vi "test_mzi_fft.vi"() -> ()   [LabVIEW 2009]
doc: "Copyright (c) 2010 Stepan A. Baranov (stepan@baranov.su)\nAll rights reserved.\nweb-site: www.OCTLab.org"
uses:
  <vilib>/Analysis/4window.llb/Hanning Window (DBL).vi
  <vilib>/Analysis/NI_AALPro.lvlib
  OCTLib_64.dll
panel:
  out "error out":errorcluster
  out "Im part":dbl[](array[numeric])
  out "Re part":dbl[](array[numeric])
  out "Phase A-scan":dbl[](array[numeric])
  out "Intensity A-scan":dbl[](array[numeric])
  out "Im":dbl[](array[numeric])
  out "Re":dbl[](array[numeric])
  out "phase":dbl[](array[numeric])
  out "intensity":dbl[](array[numeric])
  out "time for FFT":u32
  in  "RSM_STAT?":bool=TRUE
  in  "stop":bool
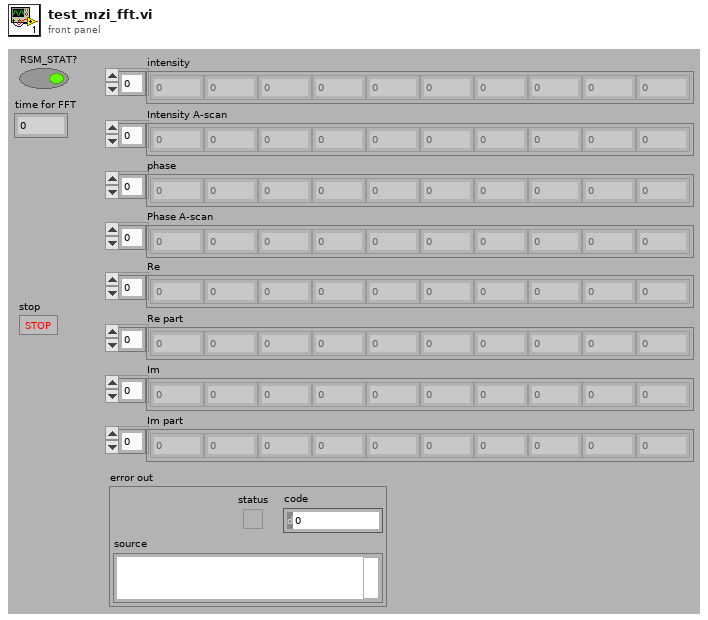
[diagram p1: front panel]
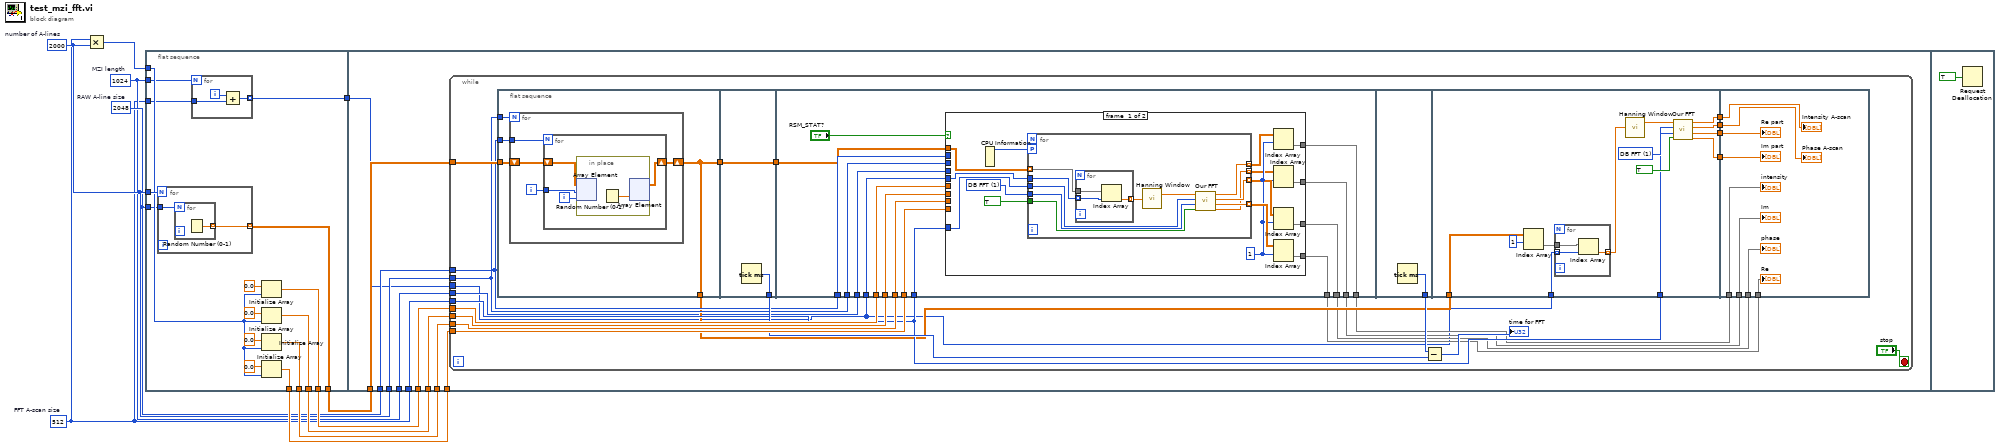
[diagram p0: block diagram]
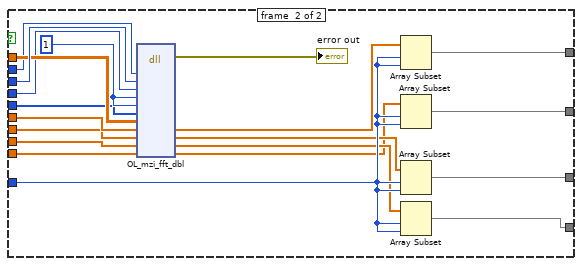
[diagram p2: hidden frame]
diagram:
  w2 = 1024  # MZI length
  w1 = 512  # FFT A-scan size
  w5 = 2000  # number of A-lines
  w4 = 2048  # RAW A-line size
  n1 = Multiply(x=w1, y=w5) -> (x*y=w11:i32)
  n2 = flat-sequence {
    tunnel: w4 -> [w15]
    tunnel: w5 -> [w26]
    tunnel: w11 -> [w21]
    tunnel: [w20] -> w10
    tunnel: [w19] -> w9
    tunnel: [w18] -> w8
    tunnel: [w17] -> w7
    tunnel: [w16] -> w6
    tunnel: [w14] -> w3
    tunnel: w2 -> [w13]
    tunnel: w1 -> [w12]
    tunnel: w5 -> [w42]
    tunnel: w4 -> [w41]
    tunnel: w10 -> [w40]
    tunnel: w9 -> [w39]
    tunnel: w8 -> [w38]
    tunnel: w7 -> [w37]
    tunnel: w6 -> [w36]
    tunnel: w1 -> [w35]
    tunnel: w3 -> [w34]
    tunnel: w2 -> [w33]
    frame #0 {
      n3 = for {
        N: w26 -> [_]
        tunnel: [w31] -> w16 mode=indexing
        tunnel: w15 -> [w30]
        n4 = for {
          N: w30 -> [_]
          tunnel: [w32] -> w31 mode=indexing
          n5 = Random Number (0-1)() -> (number: 0 to 1=w32:dbl)
        }
      }
      n6 = for {
        N: w13 -> [_]
        tunnel: [w27] -> w14 mode=indexing
        tunnel: w12 -> [w29]
        i -> [w28]
        n7 = Add(x=w28, y=w29) -> (x+y=w27:i32)
      }
      n8 = Initialize Array(0.0 ("element"), w21) -> (w19:dbl[])
      n9 = Initialize Array(0.0 ("element"), w21) -> (w18:dbl[])
      n10 = Initialize Array(0.0 ("element"), w21) -> (w20:dbl[])
      n11 = Initialize Array(0.0 ("element"), w21) -> (w17:dbl[])
    }
    frame #1 {
      n12 = while {
        tunnel: w36 -> [w66]
        tunnel: w42 -> [w58]
        tunnel: w41 -> [w57]
        tunnel: w40 -> [w65]
        tunnel: w39 -> [w64]
        tunnel: w38 -> [w63]
        tunnel: w37 -> [w62]
        tunnel: w35 -> [w56]
        tunnel: w34 -> [w43]
        tunnel: w33 -> [w44]
        stop <- "stop" stop-if-true
        n13 = flat-sequence {
          tunnel: w66 -> [w71]
          tunnel: w58 -> [w70]
          tunnel: w57 -> [w69]
          tunnel: [w68] -> w55
          tunnel: [w68] -> w45
          tunnel: [w82] -> w61
          tunnel: [w81] -> w46
          tunnel: w45 -> [w81]
          tunnel: w65 -> [w96]
          tunnel: w64 -> [w95]
          tunnel: w63 -> [w94]
          tunnel: w62 -> [w93]
          tunnel: w57 -> [w92]
          tunnel: w58 -> [w91]
          tunnel: [w90] -> w50
          tunnel: [w89] -> w49
          tunnel: [w88] -> w48
          tunnel: [w87] -> w47
          tunnel: w56 -> [w86]
          tunnel: w46 -> [w85]
          tunnel: w43 -> [w84]
          tunnel: w44 -> [w83]
          tunnel: [w147] -> w59
          tunnel: w55 -> [w160]
          tunnel: w56 -> [w155]
          tunnel: [w154] -> w54
          tunnel: [w153] -> w53
          tunnel: [w152] -> w52
          tunnel: [w151] -> w51
          tunnel: w43 -> [w150]
          tunnel: w54 -> [w171]
          tunnel: w53 -> [w170]
          tunnel: w52 -> [w169]
          tunnel: w51 -> [w168]
          tunnel: w50 -> [w167]
          tunnel: w49 -> [w166]
          tunnel: w48 -> [w165]
          tunnel: w47 -> [w164]
          frame #0 {
            n14 = for {
              N: w70 -> [_]
              shift-right: [w73] -> w68
              shift-left: w71 -> [w74]
              tunnel: w69 -> [w75]
              i -> [w72]
              n15 = for {
                N: w75 -> [_]
                shift-right: [w76] -> w73
                shift-left: w74 -> [w79]
                tunnel: w72 -> [w78]
                i -> [w77]
                n16 = in-place {
                  n17 = in-place-array #1(w79, w78, w77) -> ()  [unwired: 1 out]
                  n18 = Random Number (0-1)() -> (number: 0 to 1=w80:dbl)
                  n19 = in-place-array #1(w80) -> (w76:dbl[][])  [unwired: 2 out]
                }
              }
            }
          }
          frame #1 {
            n20 = Tick Count (ms)() -> (millisecond timer value=w82:u32)
          }
          frame #2 {
            n21 = case shown="True" "RSM_STAT?" {
              tunnel: w96 -> [_ w143]
              tunnel: w95 -> [_ w146]
              tunnel: w94 -> [_ w145]
              tunnel: w93 -> [_ w144]
              tunnel: w92 -> [_ w130]
              tunnel: w91 -> [_ w142]
              tunnel: w85 -> [w112 w140]
              tunnel: [w109 w138] -> w90
              tunnel: [w107 w135] -> w89
              tunnel: [w106 w133] -> w88
              tunnel: [w103 w131] -> w87
              tunnel: w86 -> [w111 w139]
              tunnel: w84 -> [w100 w129]
              tunnel: w83 -> [_ w128]
              frame #0 {
                w98 = 1 items=["LINEAR FFT", "DB FFT"] ("A-scan type")
                w104 = 1 ("index (row)")
                n22 = CPU Information() -> (4:w101:i32)  [unwired: 3 out]
                n23 = for {
                  workers-P: w101 -> [_]
                  tunnel: [w122] -> w110 mode=indexing
                  tunnel: [w121] -> w108 mode=indexing
                  tunnel: [w120] -> w105 mode=indexing
                  tunnel: [w119] -> w102 mode=indexing
                  tunnel: w112 -> [w116] mode=indexing
                  tunnel: w111 -> [w118]
                  tunnel: w100 -> [w117]
                  tunnel: TRUE ("need phase?") -> [w114]
                  tunnel: w98 -> [w113]
                  n24 = for {
                    tunnel: w117 -> [w125] mode=indexing
                    tunnel: w116 -> [w126]
                    tunnel: [w124] -> w115 mode=indexing
                    n25 = Index Array(array=w126, index=w125) -> (element=w124:dbl)
                  }
                  n26 = call-poly <vilib>:"Hanning Window.vi"("X"=w115) -> ("Windowed X"=w123:dbl[])  [unwired: 1 out]
                  n27 = call "Our FFT.vi"("need phase?"=w114, "A-scan type"=w113, "FFT A-scan size"=w118, "RAW A-line"=w123) -> ("Im part"=w119:dbl[], "Re part"=w120:dbl[], "Phase A-scan"=w121:dbl[], "Intensity A-scan"=w122:dbl[])
                }
                n28 = Index Array(array=w110, index (row)=w104) -> (element=w109:dbl[])  [unwired: 1 in]
                n29 = Index Array(array=w102, index (row)=w104) -> (element=w103:dbl[])  [unwired: 1 in]
                n30 = Index Array(array=w108, index (row)=w104) -> (element=w107:dbl[])  [unwired: 1 in]
                n31 = Index Array(array=w105, index (row)=w104) -> (element=w106:dbl[])  [unwired: 1 in]
              }
              frame #1 {
                w141 = i8 1 ("hanning_flag")
                n32 = dll-call lib="OCTLib**.*" fn="OL_mzi_fft_dbl"("width"=w130, "height"=w142, "mzi_length"=w128, "hanning_flag"=w141, "log10_flag"=w141, "mzi_indexes"=w129, "input"=w140, "intensity"=w146, "phase"=w145, "Re"=w143, "Im"=w144) -> (error out=→"error out":errorcluster, "intensity"=w137:dbl[], "phase"=w136:dbl[], "Re"=w134:dbl[], "Im"=w132:dbl[])  [unwired: 11 in, 1 out]
                n33 = Array Subset(array=w137, index=w139, length=w139) -> (w138:dbl[])
                n34 = Array Subset(array=w132, index=w139, length=w139) -> (w131:dbl[])
                n35 = Array Subset(array=w136, index=w139, length=w139) -> (w135:dbl[])
                n36 = Array Subset(array=w134, index=w139, length=w139) -> (w133:dbl[])
              }
            }
          }
          frame #3 {
            n37 = Tick Count (ms)() -> (millisecond timer value=w147:u32)
          }
          frame #4 {
            w157 = 1 items=["LINEAR FFT", "DB FFT"] ("A-scan type")
            n38 = Index Array(array=w160, index (row)=1) -> (element=w149:dbl[])  [unwired: 1 in]
            n39 = for {
              tunnel: w150 -> [w162] mode=indexing
              tunnel: w149 -> [w163]
              tunnel: [w161] -> w148 mode=indexing
              n40 = Index Array(array=w163, index=w162) -> (element=w161:dbl)
            }
            n41 = call-poly <vilib>:"Hanning Window.vi"("X"=w148) -> ("Windowed X"=w158:dbl[])  [unwired: 1 out]
            n42 = call "Our FFT.vi"("need phase?"=TRUE, "A-scan type"=w157, "FFT A-scan size"=w155, "RAW A-line"=w158) -> ("Im part"=w151:dbl[], "Re part"=w152:dbl[], "Phase A-scan"=w153:dbl[], "Intensity A-scan"=w154:dbl[])
          }
          frame #5 {
            "Intensity A-scan" <- w171
            "Phase A-scan" <- w170
            "Re part" <- w169
            "Im part" <- w168
            "intensity" <- w167
            "phase" <- w166
            "Re" <- w165
            "Im" <- w164
          }
        }
        n43 = Subtract(x=w59, y=w61) -> (x-y=→"time for FFT":u32)
      }
    }
    frame #2 {
      n44 = Request Deallocation(TRUE ("flag")) -> ()
    }
  }
